vi "GetDeviceList.vi"(8 "error in (no error)":errorcluster, 10 "Dev Type":i32, 11 "Combo Box":refnum<vi>) -> (0 "error out":errorcluster, 3 "Current Selection":string)   [LabVIEW 2009]
doc: "GetSCDsFromReg.vi\n\nUsed to retrieve the list of all currently registered devices by type and prepare them for display in a combo box.\n\n\nInputs - \nCombo Box - this is a reference to the combo box that will contain the list \n of Devices\n\nDev Type - Device Type code\n MCD = 1\n SCD = 2\n Mono = 3\n FW = 4\n Polarizer = 5\n Temperature Controller = 6\n \nError In - Input Error cluster\n\n---------------------------\nOutputs -\nCurrent Selection - Display name of first SCD in the list. Use this as an\n input to the Val(Sgnl) property of the combo box to\n make this the current selection\n\n\nError Out - Output Error cluster"
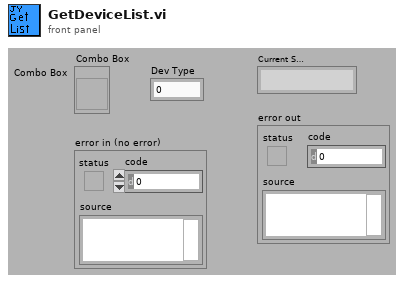
[diagram p1: front panel]
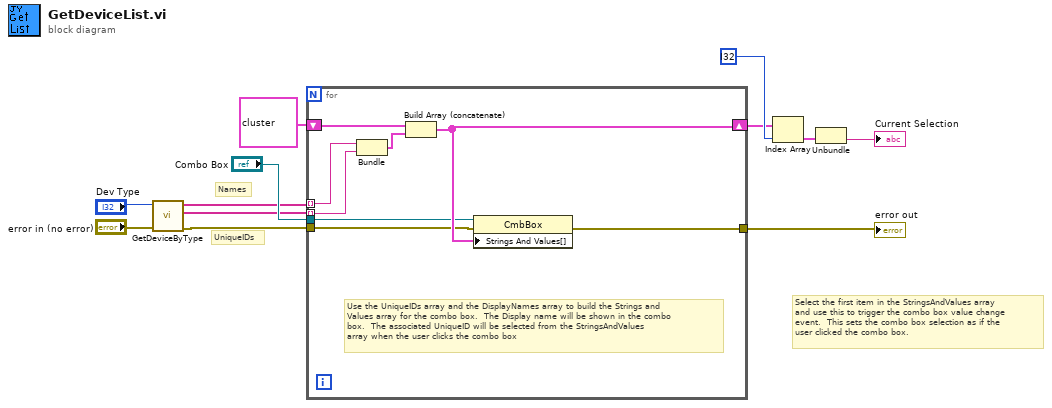
[diagram p0: block diagram]
diagram:
  # "UniqueIDs"
  # "Names"
  # "Select the first item in the StringsAndValues array\nand use this to trigger the combo box value change\nevent.  This sets the combo box selection as if the\nuser clicked the combo box."
  n1 = call "GetDeviceByType.vi"("error in (no error)"="error in (no error)", "DevType"="Dev Type") -> ("error out"=w3:errorcluster, "UniqueIDs"=w2:string[], "Names"=w1:string[])  [unwired: 7 out]
  n2 = for {
    tunnel: w1 -> [w20] mode=indexing
    tunnel: w2 -> [w19] mode=indexing
    shift-right: [w16] -> w10
    shift-left: cluster{"String":string, "String":string}[] ? -> [w17]
    tunnel: w3 -> [w15]
    tunnel: [w14] -> w6
    tunnel: "Combo Box" -> [w13]
    # "Use the UniqueIDs array and the DisplayNames array to build the Strings and\nValues array for the combo box.  The Display name will be shown in the combo\nbox.  The associated UniqueID will be selected from the StringsAndValues \narray when the user clicks the combo box"
    n3 = Bundle("String"=w20, "String"=w19) -> (w18:cluster{"String":string, "String":string})  [unwired: 1 out]
    n4 = Build Array (concatenate)(w17, w18) -> (w16:cluster{"String":string, "String":string}[])
    n5 = property on="Property Node" class="CmbBox"(reference=w13, error in=w15, "Strings And Values[]"=w16) -> (error out=w14:errorcluster)  [unwired: 1 out]
  }
  "error out" <- w6
  n6 = Index Array(array=w10, index=i32 ?) -> (element=w12:cluster{"String":string, "String":string})
  n7 = Unbundle(w12) -> ("String"=→"Current Selection":string)  [unwired: 1 out]
